vi "VerifyArguments.vi"(8 "error in (no error)":errorcluster, 11 "SetConditionalSymbol in":refnum<class "SetConditionalSymbol.lvclass">) -> (0 "error out":errorcluster, 3 "SetConditionalSymbol out":refnum<class "SetConditionalSymbol.lvclass">)   [LabVIEW 2014, in "SetConditionalSymbol.lvclass"]
doc: "Ensures required arguments are provided to the LabVIEWCLI."
uses:
  SetConditionalSymbol.lvclass
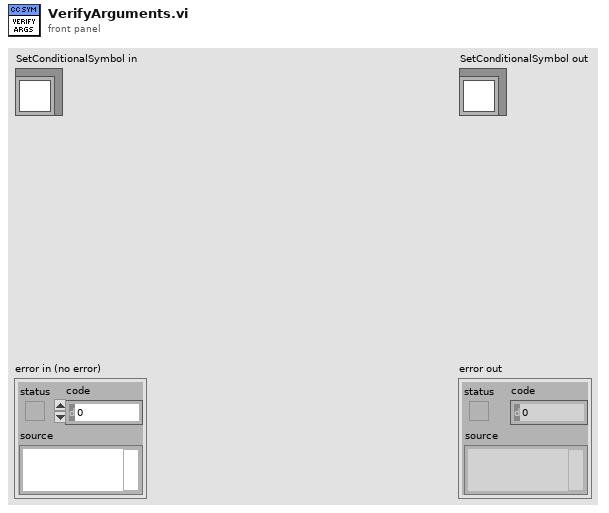
[diagram p1: front panel]
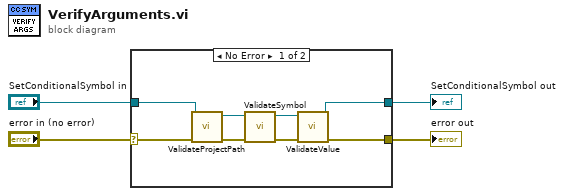
[diagram p0: block diagram]
diagram:
  n1 = case shown="No Error" "error in (no error)" {
    selector: "error in (no error)" -> [w8 w14]
    tunnel: [w7 w14] -> w3
    tunnel: [w5 w13] -> w1
    tunnel: "SetConditionalSymbol in" -> [w6 w13]
    frame No Error {
      n2 = call "ValidateProjectPath.vi"("error in (no error)"=w8, "SetConditionalSymbol in"=w6) -> ("error out"=w12:errorcluster, "SetConditionalSymbol out"=w10:refnum<class "SetConditionalSymbol.lvclass">)  [unwired: 8 in]
      n3 = call "ValidateSymbol.vi"("error in (no error)"=w12, "SetConditionalSymbol in"=w10) -> ("error out"=w11:errorcluster, "SetConditionalSymbol out"=w9:refnum<class "SetConditionalSymbol.lvclass">)  [unwired: 8 in]
      n4 = call "ValidateValue.vi"("error in (no error)"=w11, "SetConditionalSymbol in"=w9) -> ("error out"=w7:errorcluster, "SetConditionalSymbol out"=w5:refnum<class "SetConditionalSymbol.lvclass">)  [unwired: 8 in]
    }
    frame Error {
    }
  }
  "error out" <- w3
  "SetConditionalSymbol out" <- w1
